vi "Write Communication Channel.vi"(8 "error in (no error)":errorcluster, 10 "Communication Channel":T1, 11 "NMR in":refnum<class "NMR.lvclass">) -> (0 "error out":errorcluster, 3 "NMR out":refnum<class "NMR.lvclass">)   [LabVIEW 2011, in "NMR.lvclass"]
uses:
  NMR.lvclass
  Communication Channel.ctl
  NMR.lvclass/NMR.ctl
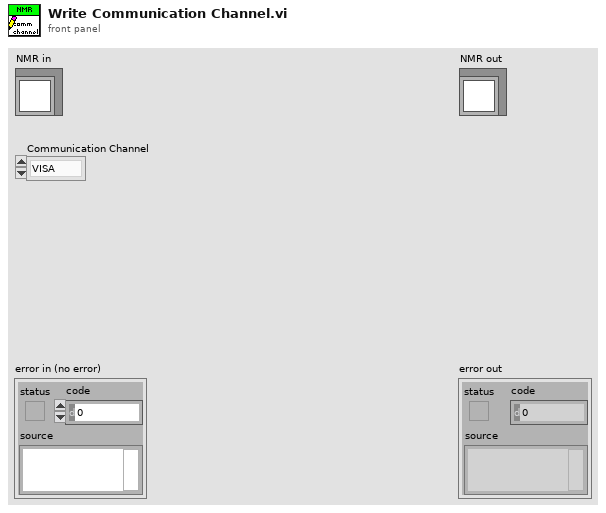
[diagram p1: front panel]
types:
  T1 = typedef "NMR.lvclass/Communication Channel.ctl" = enum16{"VISA", "DLL"}
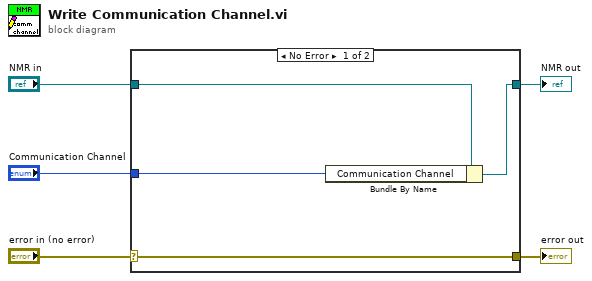
[diagram p0: block diagram]
diagram:
  n1 = case shown="No Error" "error in (no error)" {
    selector: "error in (no error)" -> [w9 w10]
    tunnel: [w9 w10] -> w4
    tunnel: [w7 w11] -> w2
    tunnel: "NMR in" -> [w8 w11]
    tunnel: "Communication Channel" -> [w6 _]
    frame No Error {
      n2 = Bundle By Name(cluster=w8, "Communication Channel"=w6) -> (w7:refnum<class "NMR.lvclass">)
    }
    frame Error {
    }
  }
  "error out" <- w4
  "NMR out" <- w2
